vi "write_do_to_db.vi"(0 "reference in":refnum<class "DO.lvclass">, 11 "error in (no error)":errorcluster) -> (4 "reference out":refnum<class "DO.lvclass">, 15 "error out":errorcluster)   [LabVIEW 2019, in "DO.lvclass"]
uses:
  DO.lvclass
  D:/GIT H4000/H4000/src/Proccess_class/Proccess.lvclass
  Proccess_class/Proccess.lvclass/Proccess.ctl
  DO.lvclass/DO.ctl
  Logger_class/Priority.ctl
  Logger_class/EventData.ctl
  Logger_class/EventCode.ctl
  Logger_class/Logger.lvclass
  Proccess_class/Proccess.lvclass
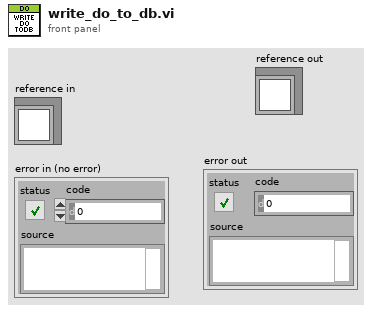
[diagram p1: front panel]
types:
  T1 = typedef "Logger.lvclass/Priority.ctl" = enum16{"Alert", "Critical", "Error", "Warning", "Notice", "Informational", "Debug"}
  T2 = typedef "Logger.lvclass/EventData.ctl" = cluster{"obj_tag":string, "event_tag":string, "code":T3, "Priority":T1, "Value":dbl, "Description":string, "Time Stamp":timestamp}
  T3 = typedef "Logger.lvclass/EventCode.ctl" = enum16{"DI_EU_LO", "DI_EU_HI", "DIO_LO", "DIO_HI", "DI_RAW_LO", "DI_RAW_HI", "DO_LO", "DO_HI", "DA_OK", "DA_ALARM", "AA_HI", "AA_HIHI", "AA_LO", "AA_LOLO", "AA_OK", "CMD", "OUT_OF_RANGE_OK", "OUT_OF_RANGE_LO", "OUT_OF_RANGE_HI", "CONFIG", "DI_LO", "DI_HI"}
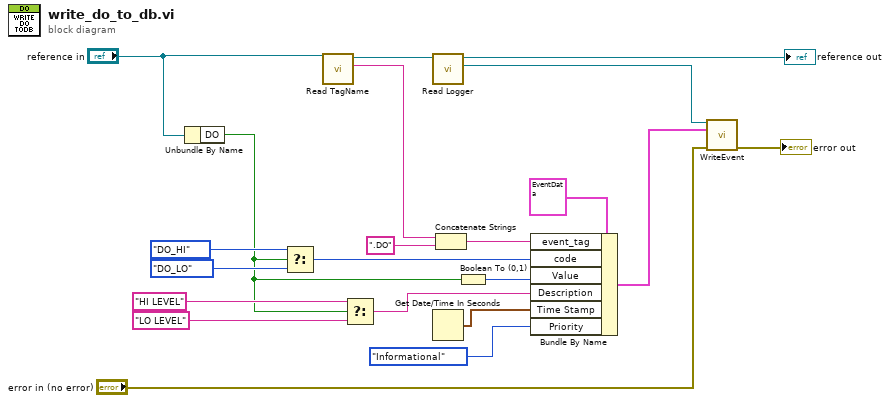
[diagram p0: block diagram]
diagram:
  n1 = Unbundle By Name("reference in") -> ("DO"=w12:bool)
  n2 = Select(t=EventCode."DO_HI" ("code"), s=w12, f=EventCode."DO_LO" ("code")) -> (s? t:f=w15:T3)
  n3 = call "Read TagName.vi"("Proccess in"="reference in") -> ("TagName"=w6:string, "Proccess out"=w5:refnum<class "DO.lvclass">)  [unwired: 9 in]
  n4 = Select(t="HI LEVEL" ("Description"), s=w12, f="LO LEVEL" ("Description")) -> (s? t:f=w10:string)
  n5 = call "Read Logger.vi"("Proccess in"=w5) -> ("Logger"=w4:refnum<class "Logger.lvclass">, "Proccess out"=→"reference out":refnum<class "DO.lvclass">)  [unwired: 9 in]
  n6 = Get Date/Time In Seconds() -> (seconds since 1Jan1904=w9:timestamp)
  n7 = Concatenate Strings(w6, ".DO" ("string")) -> (w18:string)
  n8 = Boolean To (0,1)(Boolean=w12) -> (0, 1=w14:i16)
  n9 = Bundle By Name(cluster=T2 {"obj_tag"="", "event_tag"="", "code"=enum."DI_RAW_LO", "Priority"=enum."Alert", "Value"=0.0, "Description"="", "Time Stamp"=timestamp(0 s since 1904-01-01)} ("Event"), "event_tag"=w18, "code"=w15, "Value"=w14, "Description"=w10, "Time Stamp"=w9, "Priority"=Priority."Informational") -> (w20:T2)
  n10 = call "WriteEvent.vi"("reference in"=w4, "Event"=w20, "error in (no error)"="error in (no error)") -> ("error out"=→"error out":errorcluster)  [unwired: 11 in, 1 out]
